vi "2Ch Interleaved Fxp to wfms.vi"(0 "reference in":refnum<class "Fcurve.lvclass">, 2 "Wfms (4in)":fxp<+/-,27,5>[](array[numeric]), 5 "error in (no error)":errorcluster, 8 "Channels Slow FPGA":T2(array[cluster])) -> (14 "reference out":refnum<class "Fcurve.lvclass">, 16 "Channels to save":T1(array[ring]), 17 "Wfms (4out)":waveform(dbl)[](array[waveform]), 19 "error out":errorcluster)   [LabVIEW 2019, in "Fcurve.lvclass"]
doc: "Gets the raw data of index 0 and 1 of the interleaved waveform channel and outputs it as an array for 2 channels"
uses:
  Fcurve.lvclass
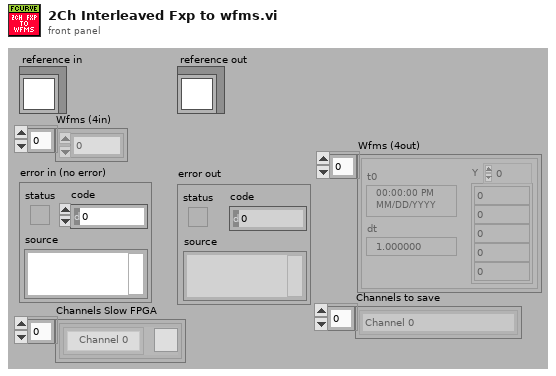
[diagram p1: front panel]
types:
  T1 = enum16{"Channel 0", "Channel 1", "Channel 2", "Channel 3"}[]
  T2 = cluster{"Channel":enum16{"Channel 0", "Channel 1", "Channel 2", "Channel 3"}, "Save?":bool}[]
  T3 = typedef "Fcurve.lvclass/ObjectAttributes.ctl" = cluster{"MyAttribute":dbl, "Fcurve Metadata":T4, "Contact Spread of dev":dbl, "Tau Delay (ms)":dbl, "Points of contact":dbl, "Def_wfm":cluster{"Max":dbl, "Min":dbl}, "Zpos_wfm":cluster{"Max":dbl, "Min":dbl}, "Contact stat?":bool, "Real AI dt (s)":dbl, "Decimation":cluster{"App":cluster{"Dec":i32, "apply":bool}, "Con":cluster{"Dec":i32, "apply":bool}, "Ret":cluster{"Dec":i32, "apply":bool}}, "Segment def[0]":dbl, "Segment Zpos[0]":dbl, "Raw Datum":waveform(dbl)[], "Group metadata":T5, "M_data obj":refnum<class "metadata.lvclass">, "Channel name(s)":string[], "Segment fcurve data":cluster{"X":dbl[], "Y":dbl[]}[], "Segment duration":cluster{"Start":i32, "Duration":i32}[], "Segment info":T6[], "Segment durations (S)":dbl[], "Segments Maxmin":T8[]}
  T4 = typedef "Fcurve.lvclass/Metadata.ctl" = cluster{"dt (us)":dbl, "Dec Factor":dbl, "Z piezo Sensitivity (nm/V)":dbl, "K (N/m)":dbl, "Sp (V)":dbl, "Contact (ms)":dbl, "Zpos contact":dbl, "Vel_app (nm/s)":dbl, "Vel_ret (nm/s)":dbl, "deltaV (nm)":dbl, "Def_V0 (v)":dbl, "Piezo gain":dbl, "invOLS (nm/V)":dbl}
  T5 = typedef "TDMS_DataHandler.lvclass/Fcurve Meta data.ctl" = cluster{"property names":string[], "property values":variant[]}
  T6 = typedef "Fcurve.lvclass/Fcurve segments --cluster.ctl" = cluster{"type":T7, "nb points":i32, "dec factor":u32, "sampling rate (S/s)":u32}
  T7 = typedef "metadata.lvclass/Segment type--combobox.ctl" = string
  T8 = typedef "Fcurve.lvclass/Segment MaxMin --cluster.ctl" = cluster{"Def":cluster{"max value":dbl, "min value":dbl}, "Zpos":cluster{"max value":dbl, "min value":dbl}}
  T9 = enum16{"Channel 0", "Channel 1", "Channel 2", "Channel 3"}
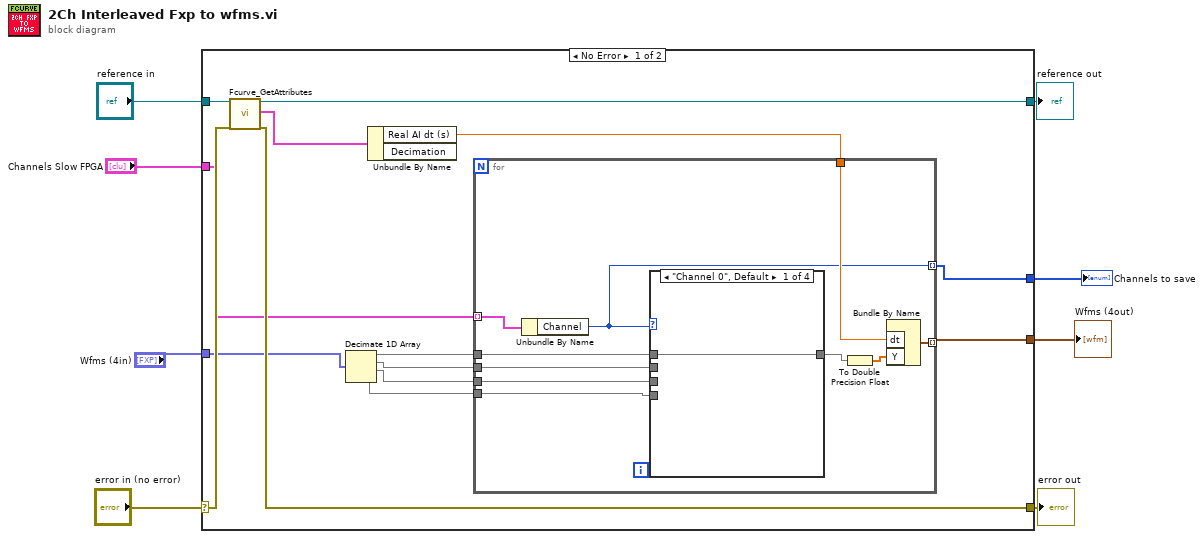
[diagram p0: block diagram]
diagram:
  n1 = case shown="No Error" "error in (no error)" {
    selector: "error in (no error)" -> [w20 w38]
    tunnel: [w19 w38] -> w7
    tunnel: [w21 w37] -> w5
    tunnel: "reference in" -> [w22 w37]
    tunnel: "Wfms (4in)" -> [w17 _]
    tunnel: "Channels Slow FPGA" -> [w11 _]
    tunnel: [w10 _] -> w2
    tunnel: [w9 _] -> w1
    frame No Error {
      n2 = call "Fcurve_GetAttributes.vi"("reference in"=w22, "error in (no error)"=w20) -> ("reference out"=w21:refnum<class "Fcurve.lvclass">, "attributes"=w18:T3, "error out"=w19:errorcluster)  [unwired: 14 in, 1 out]
      n3 = Decimate 1D Array(w17) -> (w16:fxp<+/-,27,5>[], w15:fxp<+/-,27,5>[], w14:fxp<+/-,27,5>[], w12:fxp<+/-,27,5>[])
      n4 = Unbundle By Name(w18) -> ("Real AI dt (s)"=w13:dbl)  [unwired: 1 out]
      n5 = for {
        tunnel: w16 -> [w32]
        tunnel: w15 -> [w31]
        tunnel: w14 -> [w30]
        tunnel: w12 -> [w29]
        tunnel: w13 -> [w26]
        tunnel: [w25] -> w10 mode=indexing
        tunnel: w11 -> [w24] mode=indexing
        tunnel: [w23] -> w9 mode=indexing
        n6 = Unbundle By Name(w24) -> ("Channel"=w23:T9)
        n7 = case shown="\"Channel 0\", Default" w23 {
          tunnel: w32 -> [w33 _ _ _]
          tunnel: w31 -> [_ w34 _ _]
          tunnel: w30 -> [_ _ w35 _]
          tunnel: w29 -> [_ _ _ w36]
          tunnel: [w33 w34 w35 w36] -> w27
          frame "Channel 0", Default {
          }
          frame "Channel 1" {
          }
          frame "Channel 2" {
          }
          frame "Channel 3" {
          }
        }
        n8 = To Double Precision Float(number=w27) -> (double precision float=w28:dbl[])
        n9 = Bundle By Name("dt"=w26, "Y"=w28) -> (w25:waveform(dbl))  [unwired: 1 in]
      }
    }
    frame Error {
    }
  }
  "error out" <- w7
  "reference out" <- w5
  "Wfms (4out)" <- w2
  "Channels to save" <- w1
